vi "Destroy Request Events.vi"(8 "error in (no error)":errorcluster) -> (0 "error out":errorcluster)   [LabVIEW 2023, in "Panther Dashboard.lvlib"]
doc: "Destroy the requests user events, even if there is an incoming error.\n\n<b>NOTE</b>: The contents of this VI are automatically generated and modified by the <b>Tools > Delacor > DQMH</b> utilities. Consider using those utilities instead of making your own modifications to this VI.\n_____\nBased on DQMH Project Template 6.1.0.94."
uses:
  Panther Dashboard.lvlib
panel:
  # "NOTE: The contents of this VI are automatically generated and modified by the Tools > Delacor > DQMH utilities. Consider using those utilities instead of making your own modifications to this VI."
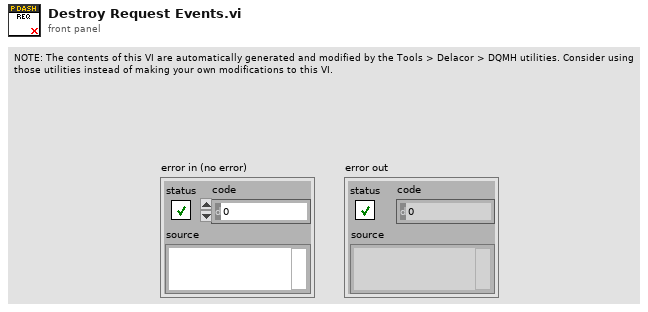
[diagram p1: front panel]
types:
  T1 = typedef "Panther Dashboard.lvlib/Request Events--cluster.ctl" = cluster{"Stop Module":refnum<user-event>, "Show Panel":refnum<user-event>, "Hide Panel":refnum<user-event>, "Get Module Execution Status":refnum<user-event>, "Show Diagram":refnum<user-event>, "Scan DQMH Modules":refnum<user-event>, "Tree DQMH Selection":refnum<user-event>, "Open Module API Tester":refnum<user-event>, "Execute Default Event Request":refnum<user-event>, "Expand Results":refnum<user-event>, "Launch DQMH Scripting Tools":refnum<user-event>, "Generate Project Documentation":refnum<user-event>, "Set App Theme":refnum<user-event>, "Show About":refnum<user-event>, "Update Module ID":refnum<user-event>, "Save Library Description":refnum<user-event>, "Save VI Description":refnum<user-event>, "Open Documentation":refnum<user-event>, "Save Project Documentation":refnum<user-event>, "Register controls Mouse Enter":refnum<user-event>, "Save Module Spec":refnum<user-event>}
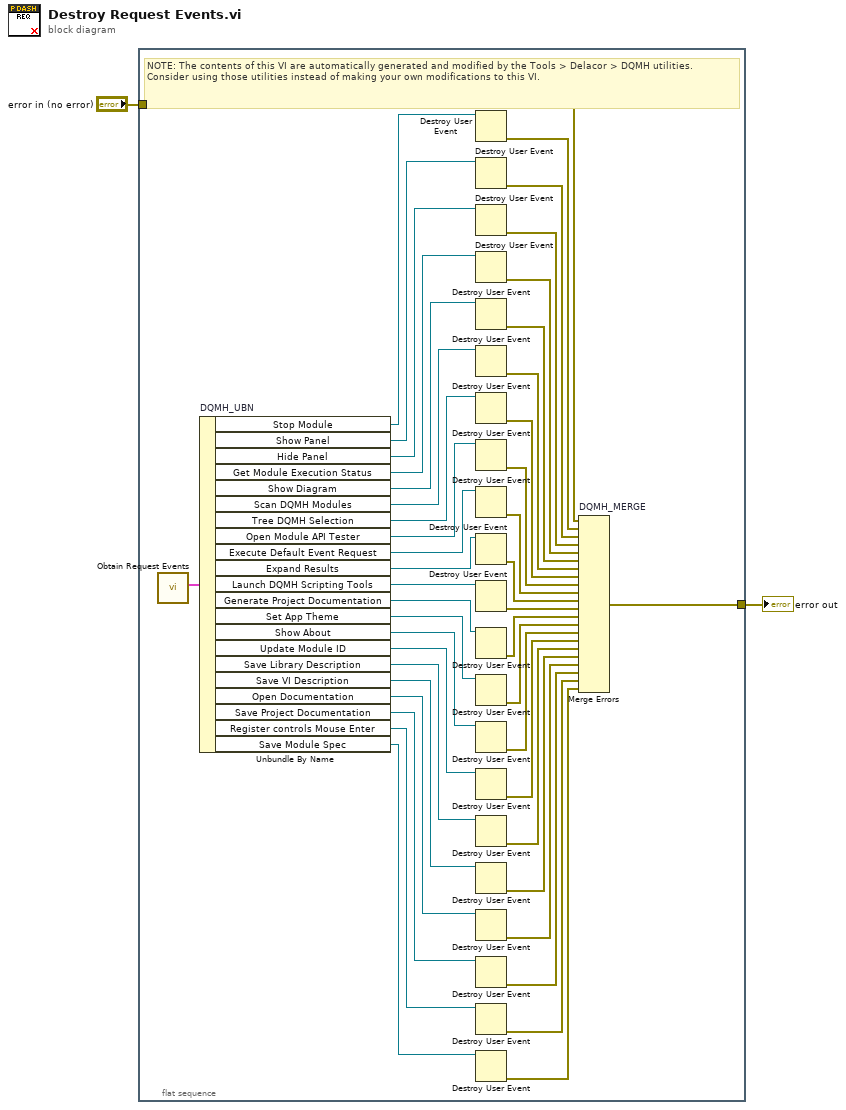
[diagram p0: block diagram]
diagram:
  n1 = flat-sequence {
    tunnel: [w46] -> w2
    tunnel: "error in (no error)" -> [w39]
    frame #0 {
      # "NOTE: The contents of this VI are automatically generated and modified by the Tools > Delacor > DQMH utilities. Consider using those utilities instead of making your own modifications to this VI."
      n2 = call "Obtain Request Events.vi"() -> ("Panther Dashboard Request Events"=w45:T1)  [unwired: 10 in, 1 out]
      n3 = Unbundle By Name "DQMH_UBN"(w45) -> ("Stop Module"=w44:refnum<user-event>, "Show Panel"=w41:refnum<user-event>, "Hide Panel"=w40:refnum<user-event>, "Get Module Execution Status"=w37:refnum<user-event>, "Show Diagram"=w35:refnum<user-event>, "Scan DQMH Modules"=w33:refnum<user-event>, "Tree DQMH Selection"=w31:refnum<user-event>, "Open Module API Tester"=w29:refnum<user-event>, "Execute Default Event Request"=w27:refnum<user-event>, "Expand Results"=w25:refnum<user-event>, "Launch DQMH Scripting Tools"=w23:refnum<user-event>, "Generate Project Documentation"=w21:refnum<user-event>, "Set App Theme"=w19:refnum<user-event>, "Show About"=w17:refnum<user-event>, "Update Module ID"=w15:refnum<user-event>, "Save Library Description"=w13:refnum<user-event>, "Save VI Description"=w11:refnum<user-event>, "Open Documentation"=w9:refnum<user-event>, "Save Project Documentation"=w7:refnum<user-event>, "Register controls Mouse Enter"=w5:refnum<user-event>, "Save Module Spec"=w3:refnum<user-event>)
      n4 = Destroy User Event(user event=w44) -> (error out=w47:errorcluster)  [unwired: 1 in]
      n5 = Destroy User Event(user event=w41) -> (error out=w43:errorcluster)  [unwired: 1 in]
      n6 = Destroy User Event(user event=w40) -> (error out=w42:errorcluster)  [unwired: 1 in]
      n7 = Destroy User Event(user event=w37) -> (error out=w38:errorcluster)  [unwired: 1 in]
      n8 = Destroy User Event(user event=w35) -> (error out=w36:errorcluster)  [unwired: 1 in]
      n9 = Destroy User Event(user event=w33) -> (error out=w34:errorcluster)  [unwired: 1 in]
      n10 = Destroy User Event(user event=w31) -> (error out=w32:errorcluster)  [unwired: 1 in]
      n11 = Destroy User Event(user event=w29) -> (error out=w30:errorcluster)  [unwired: 1 in]
      n12 = Destroy User Event(user event=w27) -> (error out=w28:errorcluster)  [unwired: 1 in]
      n13 = Destroy User Event(user event=w25) -> (error out=w26:errorcluster)  [unwired: 1 in]
      n14 = Destroy User Event(user event=w23) -> (error out=w24:errorcluster)  [unwired: 1 in]
      n15 = Destroy User Event(user event=w21) -> (error out=w22:errorcluster)  [unwired: 1 in]
      n16 = Destroy User Event(user event=w19) -> (error out=w20:errorcluster)  [unwired: 1 in]
      n17 = Destroy User Event(user event=w17) -> (error out=w18:errorcluster)  [unwired: 1 in]
      n18 = Destroy User Event(user event=w15) -> (error out=w16:errorcluster)  [unwired: 1 in]
      n19 = Destroy User Event(user event=w13) -> (error out=w14:errorcluster)  [unwired: 1 in]
      n20 = Destroy User Event(user event=w11) -> (error out=w12:errorcluster)  [unwired: 1 in]
      n21 = Destroy User Event(user event=w9) -> (error out=w10:errorcluster)  [unwired: 1 in]
      n22 = Destroy User Event(user event=w7) -> (error out=w8:errorcluster)  [unwired: 1 in]
      n23 = Destroy User Event(user event=w5) -> (error out=w6:errorcluster)  [unwired: 1 in]
      n24 = Destroy User Event(user event=w3) -> (error out=w4:errorcluster)  [unwired: 1 in]
      n25 = Merge Errors "DQMH_MERGE"(w39, w47, w43, w42, w38, w36, w34, w32, w30, w28, w26, w24, w22, w20, w18, w16, w14, w12, w10, w8, w6, w4) -> (w46:errorcluster)
    }
  }
  "error out" <- w2
